vi "Calculate_steering_motor.vi"(8 "Invert?":bool, 9 "Offset Angle":dbl(knob) scale=-180.0..180.0, 10 "Absolute Position":dbl, 11 "Angle":dbl(knob) scale=-180.0..180.0) -> (0 "Position corrected":dbl, 3 "Steering Motor Output":dbl format="%.2f")   [LabVIEW 2023]
uses:
  <vilib>/addons/control/pid/pid.llb/PID (DBL).vi
  <vilib>/addons/control/pid/NI_PID_pid.lvlib
panel:
  out "angle error (scaled)":dbl
  in  "PID gains":T1={"proportional gain (Kc)"=1.0, "integral time (Ti, min)"=0.01, "derivative time (Td, min)"=0.0} {"derivative time (Td, min)" format="%.3f"; "integral time (Ti, min)" format="%.3f"; "proportional gain (Kc)" format="%.3f"}
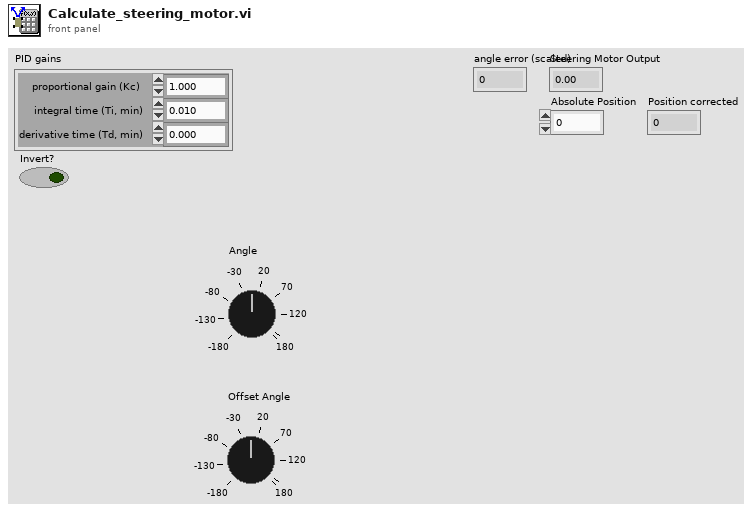
[diagram p1: front panel]
types:
  T1 = cluster{"proportional gain (Kc)":dbl, "integral time (Ti, min)":dbl, "derivative time (Td, min)":dbl}
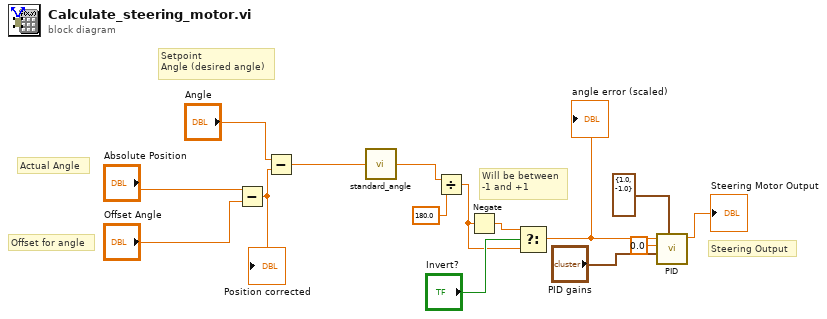
[diagram p0: block diagram]
diagram:
  # "Steering Output"
  # "Will be between\n-1 and +1"
  # "Offset for angle"
  # "Actual Angle"
  # "Setpoint\nAngle (desired angle)"
  n1 = Subtract(x="Absolute Position", y="Offset Angle") -> (x-y=w9:dbl)
  "Position corrected" <- w9
  n2 = Subtract(x="Angle", y=w9) -> (x-y=w2:dbl)
  n3 = call "standard_angle.vi"("angle in"=w2) -> ("angle out"=w1:dbl)
  n4 = Divide(x=w1, y=180.0) -> (x/y=w4:dbl)
  n5 = Negate(x=w4) -> (-x=w7:dbl)
  n6 = Select(t=w7, s="Invert?", f=w4) -> (s? t:f=w5:dbl)
  "angle error (scaled)" <- w5
  n7 = call-poly <vilib>:"PID.vi"("output range"=cluster{"output high":dbl, "output low":dbl} {"output high"=1.0, "output low"=-1.0}, "PID gains"="PID gains", "process variable"=0.0, "setpoint"=w5) -> ("output"=→"Steering Motor Output":dbl)  [unwired: 6 in, 1 out]
